vi "update.vi"(8 "error in (no error)":errorcluster, 11 "ClockDL090202FPGA in":refnum<class "ClockDL090202FPGA.lvclass">) -> (0 "error out":errorcluster, 3 "ClockDL090202FPGA out":refnum<class "ClockDL090202FPGA.lvclass">)   [LabVIEW 2010, in "ClockDL090202FPGA.lvclass"]
uses:
  ClockDL090202FPGA.lvclass
  ClockDL090202FPGA.lvclass/ClockDL090202FPGA.ctl
  GenericClock/GenericClock/GenericClock.lvclass
  FPGAWrapper/GenericFPGAWrapper/GenericFPGAWrapper/GenericFPGAWrapper.lvclass
  common/classes/GenericComponent/GenericComponent/class_data.vi
  common/classes/ErrorController/ErrorController/class_data.vi
  common/classes/GenericComponent/GenericComponent/GenericComponent.lvclass
  common/classes/ErrorController/ErrorController/ErrorController.lvclass
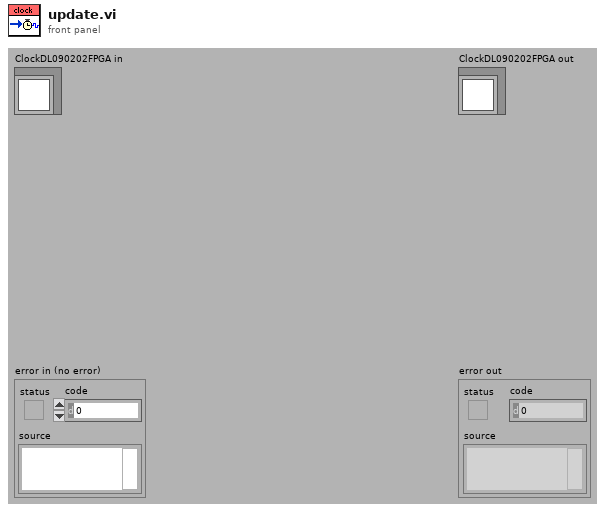
[diagram p1: front panel]
types:
  T1 = typedef "ClockDL090202FPGA.lvclass/type_enum.ctl" = enum16{"pixel clock", "gate 1", "gate 2", "gate 3"}
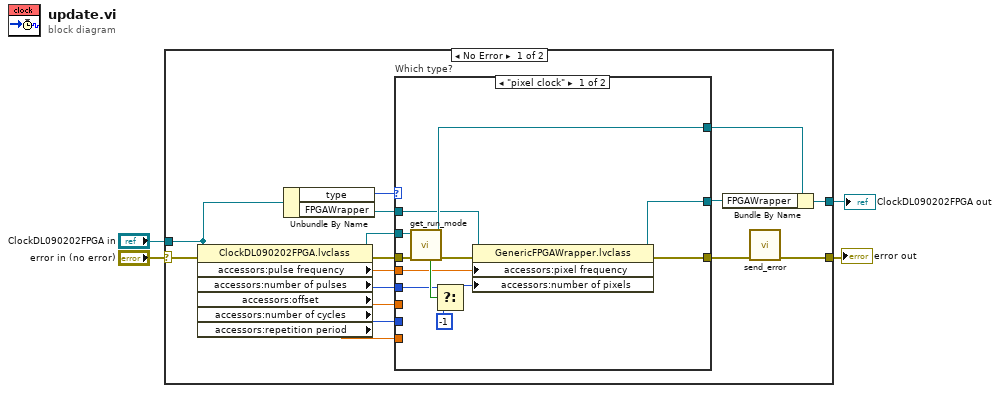
[diagram p0: block diagram]
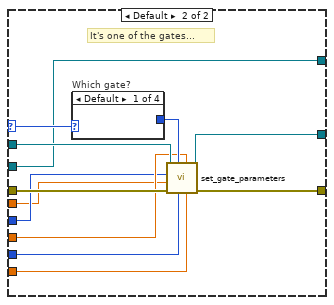
[diagram p2: hidden frame]
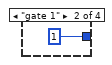
[diagram p3: hidden frame]
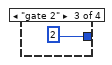
[diagram p4: hidden frame]
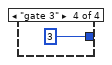
[diagram p5: hidden frame]
diagram:
  n1 = case shown="No Error" "error in (no error)" {
    selector: "error in (no error)" -> [w14 w49]
    tunnel: [w16 w49] -> w4
    tunnel: [w17 w48] -> w3
    tunnel: "ClockDL090202FPGA in" -> [w9 w48]
    frame No Error {
      n2 = property class="ClockDL090202FPGA.lvclass"(reference=w9, error in=w14) -> (reference out=w12:refnum<class "ClockDL090202FPGA.lvclass">, error out=w11:errorcluster, "accessors:pulse frequency"=w8:dbl[unit], "accessors:number of pulses"=w7:i64, "accessors:offset"=w13:dbl[unit], "accessors:number of cycles"=w6:i64, "accessors:repetition period"=w5:dbl[unit])
      n3 = Unbundle By Name(w9) -> ("type"=w19:T1, "FPGAWrapper"=w10:refnum<class "GenericFPGAWrapper.lvclass">)
      n4 = case "Which type?" shown="\"pixel clock\"" w19 {
        selector: w19 -> [_ w42]
        tunnel: w10 -> [w27 w40]
        tunnel: w11 -> [w29 w39]
        tunnel: [w22 w44] -> w15
        tunnel: [w21 w43] -> w20
        tunnel: w12 -> [w31 w38]
        tunnel: [w28 w38] -> w18
        tunnel: w13 -> [_ w37]
        tunnel: w7 -> [w24 w36]
        tunnel: w8 -> [w25 w35]
        tunnel: w6 -> [_ w33]
        tunnel: w5 -> [_ w34]
        frame "pixel clock" {
          n5 = call "get_run_mode.vi"("error in (no error)"=w29, "GenericPlugin in"=w31) -> ("error out"=w26:errorcluster, "GenericPlugin out"=w28:refnum<class "ClockDL090202FPGA.lvclass">, "is NOT free run?"=w30:bool)  [unwired: 5 in, 2 out]
          n6 = Select(t=w24, s=w30, f=i64 -1 ("t")) -> (s? t:f=w23:i64)
          n7 = property class="GenericFPGAWrapper.lvclass"(reference=w27, error in=w26, "accessors:pixel frequency"=w25, "accessors:number of pixels"=w23) -> (reference out=w21:refnum<class "GenericFPGAWrapper.lvclass">, error out=w22:errorcluster)
        }
        frame Default {
          # "It's one of the gates..."
          n8 = case "Which gate?" shown="Default" w42 {
            tunnel: [_ 1 2 3] -> w41
            frame Default {
            }
            frame "gate 1" {
            }
            frame "gate 2" {
            }
            frame "gate 3" {
            }
          }
          n9 = call-dynamic "set_gate_parameters.vi"("repetition period"=w34, "offset"=w37, "number of repetitions"=w33, "clock index"=w41, "error in (no error)"=w39, "pulsing frequency"=w35, "number of pulses"=w36, "GenericFPGAWrapper in"=w40) -> ("error out"=w44:errorcluster, "GenericFPGAWrapper out"=w43:refnum<class "GenericFPGAWrapper.lvclass">)  [unwired: 2 out]
        }
      }
      n10 = Bundle By Name(cluster=w18, "FPGAWrapper"=w20) -> (w17:refnum<class "ClockDL090202FPGA.lvclass">)
      n11 = call "send_error.vi"("error in (no error)"=w15) -> ("error out"=w16:errorcluster)  [unwired: 10 in]
    }
    frame Error {
    }
  }
  "error out" <- w4
  "ClockDL090202FPGA out" <- w3
